vi "Frequency Response Function (Mag-Phase) 1-1.vi"(0 "time signal X":waveform(dbl), 1 "restart averaging (F)":bool, 2 "window parameter":dbl=nan, 5 "time signal Y":waveform(dbl), 7 "window":T1=1 items=["Rectangle"=0, "Hanning"=1, "Hamming"=2, "Blackman-Harris"=3, "Exact Blackman"=4, "Blackman"=5, "Flat Top"=6, "4 Term B-Harris "=7, "7 Term B-Harris"=8, "Low Sidelobe"=9, "Blackman Nuttall"=11, "Triangle"=30, "Bartlett-Hanning"=31, "Bohman"=32, "Parzen"=33, "Welch"=34, "Kaiser"=60, "Dolph-Chebyshev"=61, "Gaussian"=62], 9 "view":T3, 11 "error in (no error)":errorcluster, 12 "averaging parameters":T2={"averaging mode"=enum."No averaging", "weighting mode"=enum."Exponential", "number of averages"=10} {"number of averages" min=1}, 13 "FRF Mode":enum16{"H1", "H2", "H3"}(ring)) -> (3 "averaging done":bool, 4 "magnitude":cluster{"f0":dbl, "df":dbl, "magnitude":dbl[]} {"magnitude" format="%.2p"; "f0" format="%0.2p"; "df" format="%0.2p"}, 6 "phase":cluster{"f0":dbl, "df":dbl, "phase":dbl[]} {"phase" format="%.2p"; "f0" format="%0.2p"; "df" format="%0.2p"}, 8 "coherence":cluster{"f0":dbl, "df":dbl, "coherence":dbl[]}, 10 "averages completed":dbl format="%.2p", 15 "error out":errorcluster)   [LabVIEW 2020, in "NI_MAPro.lvlib"]
doc: "Computes the frequency response and the coherence based on the input signals. Results are returned as <B>magnitude</B>, <B>phase</B>, and <B>coherence</B>."
uses:
  NI_MAPro.lvlib
  windowTd.ctl
  2-chan State.ctl
  NI_AALPro.lvlib
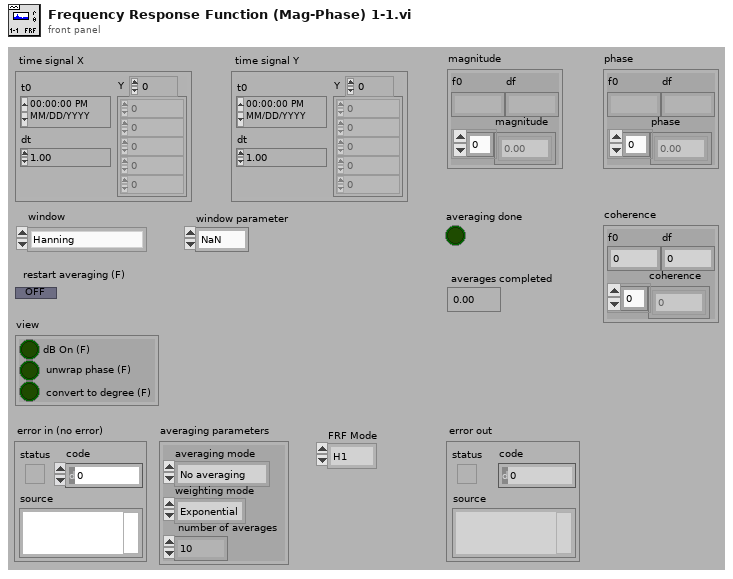
[diagram p1: front panel]
types:
  T1 = typedef "NI_AALPro.lvlib/windowTd.ctl" = u32
  T2 = cluster{"averaging mode":enum16{"No averaging", "Vector averaging", "RMS averaging", "Peak hold"}, "weighting mode":enum16{"Linear", "Exponential"}, "number of averages":u32}
  T3 = cluster{"dB On (F)":bool, "unwrap phase (F)":bool, "convert to degree (F)":bool}
  T4 = typedef "NI_MAPro.lvlib/2-chan State.ctl" = cluster{"Sx":cdb[], "Sy":cdb[], "Sxx":dbl[], "Syy":dbl[], "Sxy":cdb[], "block size":i32, "df":dbl, "dt":dbl, "avgs completed":dbl, "spectrum parameters":cluster{"averaging parameters":cluster{"averaging mode":enum16{"No averaging", "Vector averaging", "RMS averaging", "Peak hold"}, "weighting mode":enum16{"Linear", "Exponential"}, "number of averages":u32}, "window":T1}, "lin avg done":bool, "t0 history":dbl, "dt history":dbl, "timestamp":dbl}
  T5 = cluster{"f0":dbl, "df":dbl, "imag or phase":dbl[]}
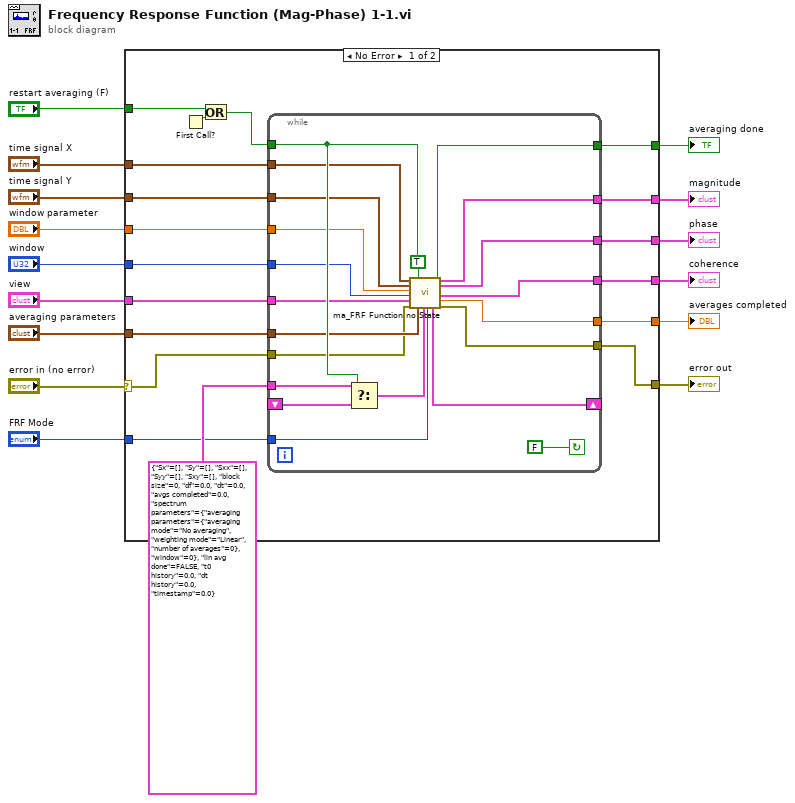
[diagram p0: block diagram]
diagram:
  n1 = case shown="No Error" "error in (no error)" {
    selector: "error in (no error)" -> [w29 w55]
    tunnel: [w30 w55] -> w14
    tunnel: "restart averaging (F)" -> [w28 _]
    tunnel: "time signal X" -> [w27 _]
    tunnel: "time signal Y" -> [w26 _]
    tunnel: "window" -> [w25 _]
    tunnel: "view" -> [w24 _]
    tunnel: "averaging parameters" -> [w23 _]
    tunnel: "FRF Mode" -> [w22 _]
    tunnel: "window parameter" -> [w21 _]
    tunnel: [w20 _] -> w5
    tunnel: [w19 _] -> w4
    tunnel: [w18 _] -> w3
    tunnel: [w17 _] -> w2
    tunnel: [w16 _] -> w1
    frame No Error {
      n2 = First Call?() -> (First Call?: T/F=w33:bool)
      n3 = Or(x=w28, y=w33) -> (x .or. y?=w31:bool)
      n4 = while {
        tunnel: w31 -> [w43]
        tunnel: [w54] -> w20
        tunnel: [w53] -> w16
        tunnel: [w52] -> w19
        tunnel: [w51] -> w30
        shift-right: [w50] -> _
        shift-left: _ -> [w47]
        tunnel: [w45] -> w18
        tunnel: T4 {"Sx"=[], "Sy"=[], "Sxx"=[], "Syy"=[], "Sxy"=[], "block size"=0, "df"=0.0, "dt"=0.0, "avgs completed"=0.0, "spectrum parameters"={"averaging parameters"={"averaging mode"=enum."No averaging", "weighting mode"=enum."Linear", "number of averages"=0}, "window"=0}, "lin avg done"=FALSE, "t0 history"=0.0, "dt history"=0.0, "timestamp"=0.0} ("state info out") -> [w44]
        tunnel: w27 -> [w42]
        tunnel: w26 -> [w41]
        tunnel: w25 -> [w40]
        tunnel: w24 -> [w39]
        tunnel: w23 -> [w38]
        tunnel: w22 -> [w37]
        tunnel: [w36] -> w17
        tunnel: w29 -> [w35]
        tunnel: w21 -> [w34]
        stop <- FALSE continue-if-true
        n5 = Select(t=w44, s=w43, f=w47) -> (s? t:f=w48:T4)
        n6 = call "ma_FRF Function no State.vi"("time signal X"=w42, "time signal Y"=w41, "window parameter"=w34, "window"=w40, "view"=w39, "error in (no error)"=w35, "restart averaging (F)"=w43, "averaging parameters"=w38, "mag-phase"=TRUE, "state info"=w48, "FRF Mode"=w37) -> ("averaging done"=w54:bool, "state info out"=w50:T4, "real or mag"=w52:cluster{"f0":dbl, "df":dbl, "real or mag":dbl[]}, "imag or phase"=w45:T5, "coherence"=w36:cluster{"f0":dbl, "df":dbl, "coherence":dbl[]}, "averages completed"=w53:dbl, "error out"=w51:errorcluster)  [unwired: 2 out]
      }
    }
    frame Error {
    }
  }
  "error out" <- w14
  "averages completed" <- w1
  "averaging done" <- w5
  "coherence" <- w2
  "magnitude" <- w4
  "phase" <- w3
